vi "rad_About Dialog.vi"() -> ()   [LabVIEW 2014]
uses:
  <vilib>/Platform/browser.llb/Open URL in Default Browser (string).vi
  rad_Globals.vi
panel:
  out "Version":string
  out "Date":string
  out "Title":string
  in  "link":bool
  in  "OK":bool
  # "Documentation and Support"
  # "NI Replication And Deployment Utility\nAugust 2012                                                                            v 2.3.01"
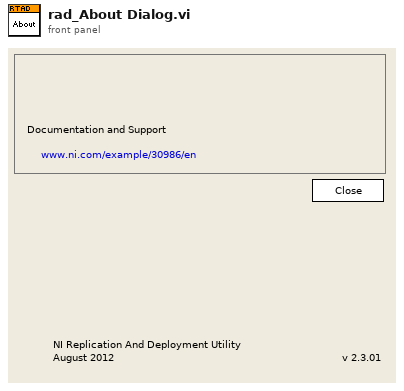
[diagram p1: front panel]
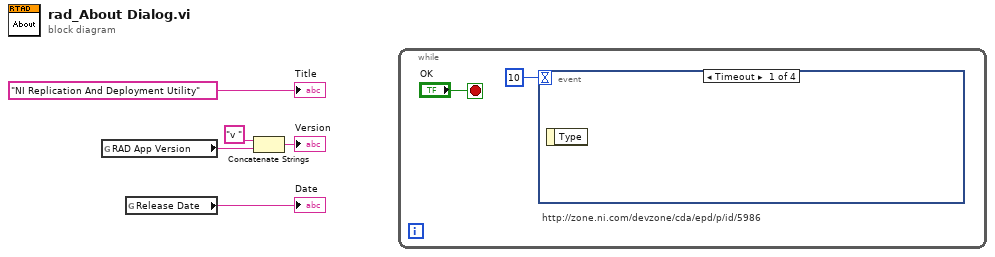
[diagram p0: block diagram]
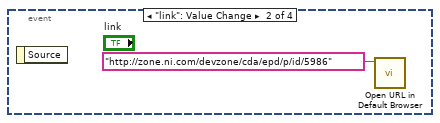
[diagram p2: hidden frame]
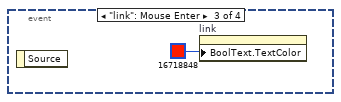
[diagram p3: hidden frame]
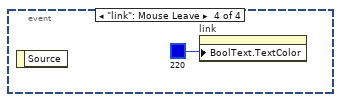
[diagram p4: hidden frame]
diagram:
  n1 = global read "rad_Globals.vi" "RAD App Version"() -> (w2:string)
  n2 = global read "rad_Globals.vi" "Release Date"() -> (→"Date":string)
  n3 = Concatenate Strings("v " ("string"), w2) -> (→"Version":string)
  n4 = while {
    stop <- "OK" stop-if-true
    # "http://zone.ni.com/devzone/cda/epd/p/id/5986"
    n5 = event shown="[0] Timeout" {
      selector: _ -> [_ _ _ _]
      dyn-events: _ -> [_ _ _ _]
      timeout: 10 -> [_ _ _ _]
      event Timeout {
        n6 = event-data() -> ()  [unwired: 1 in, 1 out]
      }
      event "link": Value Change {
        n7 = event-data() -> ()  [unwired: 1 in, 1 out]
        n8 = call-poly <vilib>:"Open URL in Default Browser.vi"("URL"="http://zone.ni.com/devzone/cda/epd/p/id/5986") -> ()  [unwired: 5 in, 2 out]
      }
      event "link": Mouse Enter {
        n9 = event-data() -> ()  [unwired: 1 in, 1 out]
        n10 = property on="link" class="Bool"("BoolText.TextColor"=u32 16718848 ("Color Box")) -> ()  [unwired: 2 in, 2 out]
      }
      event "link": Mouse Leave {
        n11 = event-data() -> ()  [unwired: 1 in, 1 out]
        n12 = property on="link" class="Bool"("BoolText.TextColor"=u32 220 ("Color Box")) -> ()  [unwired: 2 in, 2 out]
      }
    }
  }
  "Title" <- "NI Replication And Deployment Utility"
